vi "sine test.vi"() -> ()   [LabVIEW 2016]
panel:
  in  "stop":bool
  out "Waveform Chart":sgl(graph)
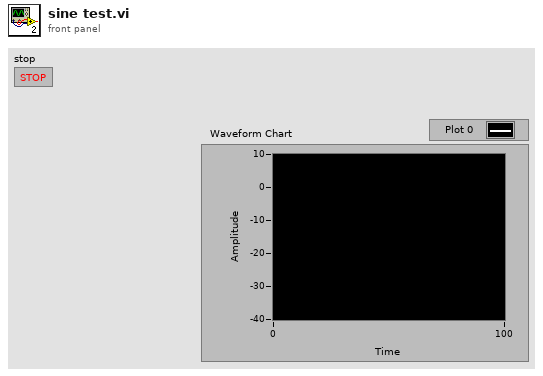
[diagram p1: front panel]
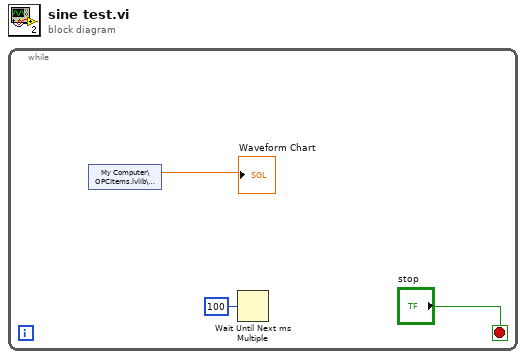
[diagram p0: block diagram]
diagram:
  n1 = while {
    stop <- "stop" stop-if-true
    n2 = shared-variable "My Computer\\OPCItems.lvlib\\Sine1"() -> (→"Waveform Chart":sgl)  [unwired: 1 in, 1 out]
    n3 = Wait Until Next ms Multiple(millisecond multiple=u32 100) -> ()  [unwired: 1 out]
  }
